vi "ComputeCenter from two straight lines.vi"(4 "delta y = 0, slope 0":bool, 5 "slope 2":dbl, 6 "intercept":dbl, 7 "intercept 2":dbl, 8 "slope":dbl, 9 "Y":sgl, 10 "X":sgl, 11 "x = 0?":bool) -> (2 "error":i32, 3 "Solution Vector":dbl[](array[numeric]))   [LabVIEW 2018]
doc: "Simply computes the intersection point of tow lines.\nBut it also handles slopes of 0 and infinity."
uses:
  <vilib>/Analysis/Matrix/Datatypes/RealMatrix.ctl
  <vilib>/Analysis/7linalg.llb/Solve Linear Equations (single right hand).vi
  <vilib>/Analysis/baseanly.llb/Solve Linear Equations By Cholesky.vi
  <vilib>/Analysis/baseanly.llb/Real Matrix to Compact Array.vi
  <vilib>/Analysis/baseanly.llb/Real Compact Tri-Matrix Linear Eqs.vi
  <vilib>/Analysis/7linalg.llb/Solve Linear Eqs (General).vi
  <vilib>/Analysis/7linalg.llb/Solve Linear Eqs (Gen, single right hand).vi
  <vilib>/Analysis/Matrix/NI_Matrix.lvlib
  <vilib>/Analysis/NI_AALPro.lvlib
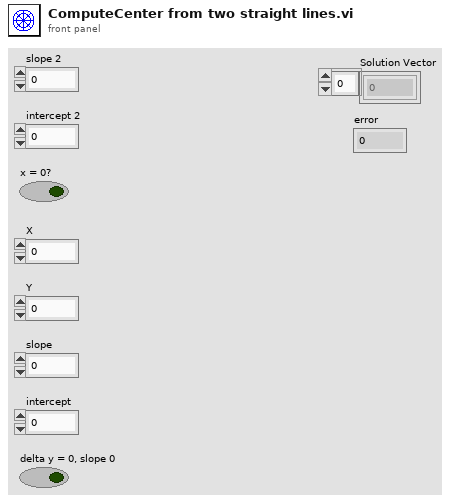
[diagram p1: front panel]
types:
  T1 = typedef "NI_Matrix.lvlib/RealMatrix.ctl" = dbl[][]
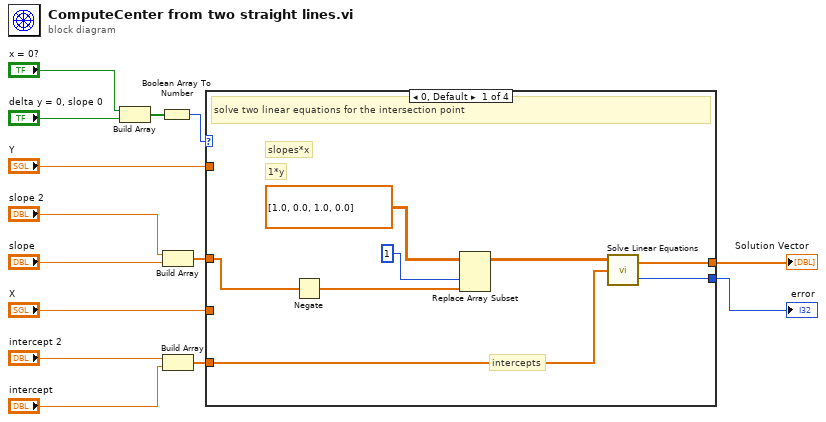
[diagram p0: block diagram]
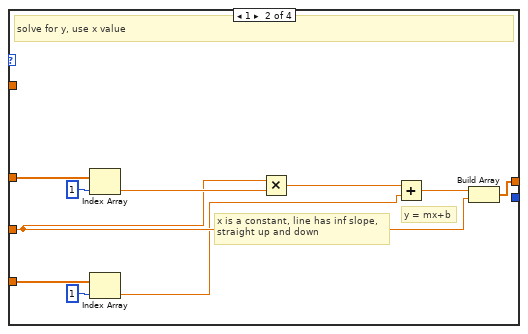
[diagram p2: hidden frame]
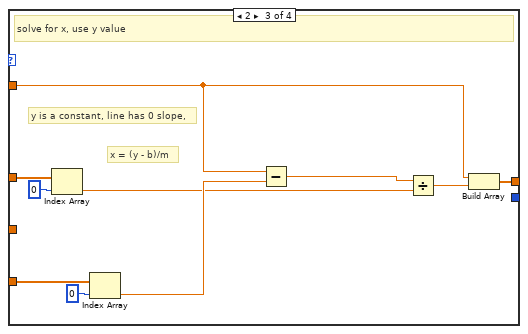
[diagram p3: hidden frame]
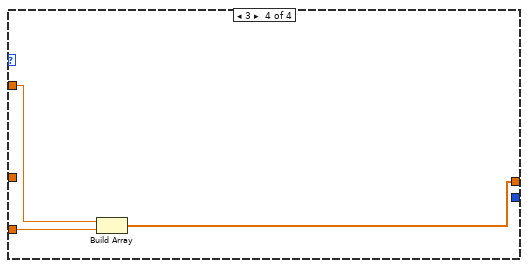
[diagram p4: hidden frame]
diagram:
  n1 = Build Array("x = 0?", "delta y = 0, slope 0") -> (w7:bool[])
  n2 = Boolean Array To Number(Boolean array=w7) -> (number=w8:u32)
  n3 = Build Array("slope 2", "slope") -> (w4:dbl[])
  n4 = Build Array("intercept 2", "intercept") -> (w2:dbl[])
  n5 = case shown="0, Default" w8 {
    tunnel: [w22 w23 w39 w43] -> w1
    tunnel: w2 -> [w21 w26 w40 _]
    tunnel: w4 -> [w18 w32 w38 _]
    tunnel: [w15 _ _ _] -> w5
    tunnel: "X" -> [_ w29 _ w44]
    tunnel: "Y" -> [_ _ w35 w45]
    frame 0, Default {
      # "intercepts"
      # "slopes*x"
      # "1*y"
      # "solve two linear equations for the intersection point"
      n6 = Negate(x=w18) -> (-x=w17:dbl[])
      n7 = Replace Array Subset(array=T1 [[1.0, 0.0], [1.0, 0.0]] ("Input Matrix"), new element=w17, index (col)=1 ("disabled index (col)")) -> (w16:T1)  [unwired: 1 in]
      n8 = call-poly <vilib>:"Solve Linear Equations.vi"("Known Vector"=w21, "Input Matrix"=w16) -> ("error"=w15:i32, "Solution Vector"=w22:dbl[])  [unwired: 1 in]
    }
    frame 1 {
      # "x is a constant, line has inf slope,\nstraight up and down"
      # "y = mx+b"
      # "solve for y, use x value"
      n9 = Index Array(array=w32, index=1) -> (element=w30:dbl)
      n10 = Index Array(array=w26, index=1) -> (element=w25:dbl)
      n11 = Multiply(x=w29, y=w30) -> (x*y=w28:dbl)
      n12 = Add(x=w28, y=w25) -> (x+y=w24:dbl)
      n13 = Build Array(w24, w29) -> (w23:dbl[])
    }
    frame 2 {
      # "y is a constant, line has 0 slope,"
      # "x = (y - b)/m"
      # "solve for x, use y value"
      n14 = Index Array(array=w38, index=0) -> (element=w34:dbl)
      n15 = Index Array(array=w40, index=0) -> (element=w37:dbl)
      n16 = Subtract(x=w35, y=w37) -> (x-y=w36:dbl)
      n17 = Divide(x=w36, y=w34) -> (x/y=w33:dbl)
      n18 = Build Array(w35, w33) -> (w39:dbl[])
    }
    frame 3 {
      n19 = Build Array(w45, w44) -> (w43:sgl[])
    }
  }
  "error" <- w5
  "Solution Vector" <- w1
